vi "Write First of Header Contents Class Array.vi"(8 "error in (no error)":errorcluster, 10 "Simulated_Header.lvclass":refnum<class "Simulated_Header.lvclass">, 11 "Save Image in":refnum<class "Save Image.lvclass">) -> (0 "error out":errorcluster, 3 "Save Image out":refnum<class "Save Image.lvclass">)   [LabVIEW 2018, in "Save Image.lvclass"]
uses:
  Save Image.lvclass
  Simulated_Header/Simulated_Header.lvclass
  Save Image.lvclass/Save Image.ctl
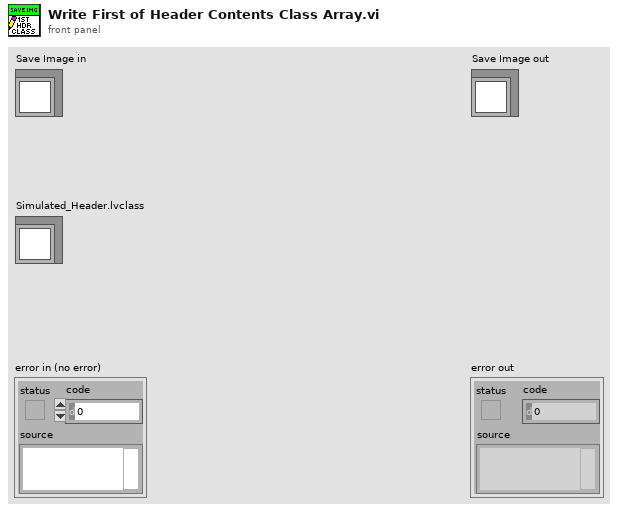
[diagram p1: front panel]
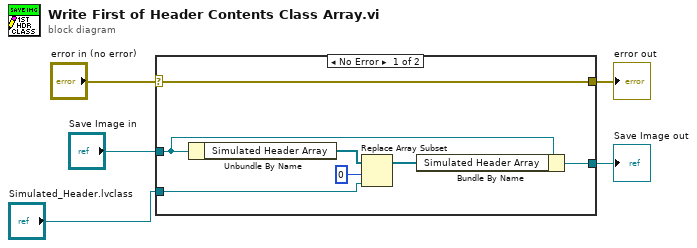
[diagram p0: block diagram]
diagram:
  n1 = case shown="No Error" "error in (no error)" {
    selector: "error in (no error)" -> [w12 w13]
    tunnel: [w12 w13] -> w4
    tunnel: [w11 w14] -> w2
    tunnel: "Save Image in" -> [w10 w14]
    tunnel: "Simulated_Header.lvclass" -> [w6 _]
    frame No Error {
      n2 = Unbundle By Name(w10) -> ("Simulated Header Array"=w9:refnum<class "Simulated_Header.lvclass">[])
      n3 = Replace Array Subset(array=w9, new element=w6, index=0) -> (w8:refnum<class "Simulated_Header.lvclass">[])
      n4 = Bundle By Name(cluster=w10, "Simulated Header Array"=w8) -> (w11:refnum<class "Save Image.lvclass">)
    }
    frame Error {
    }
  }
  "error out" <- w4
  "Save Image out" <- w2
